vi "Select Matlab if Labview Negative.vi"(8 "error in (no error)":errorcluster, 9 "Name":string, 10 "Array":cluster{"Name":string, "Data":variant}[](array[cluster]), 11 "LV value":dbl) -> (0 "error out":errorcluster, 3 "Selected value":dbl)   [LabVIEW 2010, in "Core SubVIs.lvlib"]
doc: "This vi selects the value in the LV value field if it is greater than or equal to zero. Otherwise it gets the value out of the the matlab parameter array."
uses:
  Core SubVIs.lvlib
  Matlab API/Matlab Param Array to DBL.vi
  Matlab API/Matlab API.lvlib
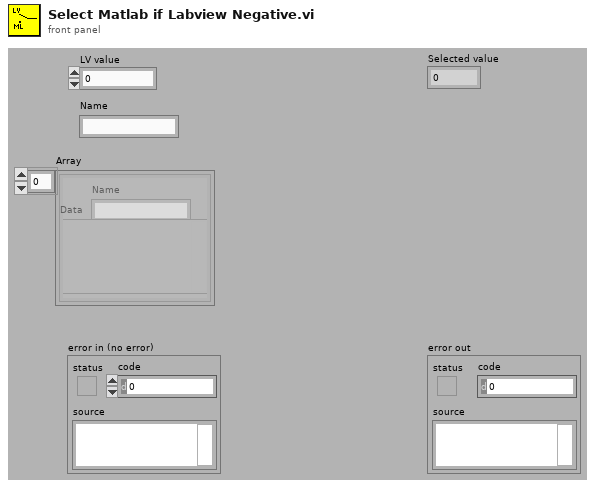
[diagram p1: front panel]
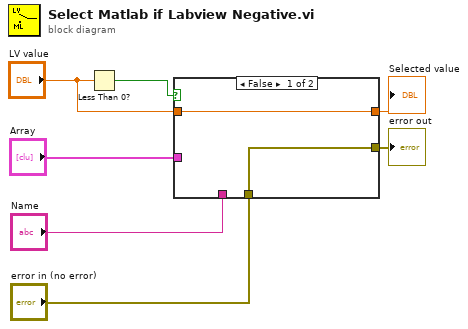
[diagram p0: block diagram]
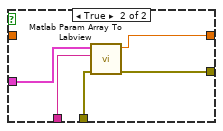
[diagram p2: hidden frame]
diagram:
  n1 = Less Than 0?(x="LV value") -> (x < 0?=w7:bool)
  n2 = case shown="False" w7 {
    tunnel: [w9 w12] -> w1
    tunnel: "LV value" -> [w9 _]
    tunnel: "Array" -> [_ w14]
    tunnel: "Name" -> [_ w13]
    tunnel: "error in (no error)" -> [w8 w11]
    tunnel: [w8 w10] -> w2
    frame False {
    }
    frame True {
      n3 = call-poly "Matlab Param Array To Labview.vi"("error in (no error)"=w11, "Name"=w13, "Matlab Param Array"=w14) -> ("error out"=w10:errorcluster, "data"=w12:dbl)  [unwired: 7 out]
    }
  }
  "error out" <- w2
  "Selected value" <- w1
